vi "Unload Subpanel VI.vi"(8 "error in":errorcluster, 11 "subpanel refnum":refnum<vi>) -> (0 "error out":errorcluster)   [LabVIEW 2010]
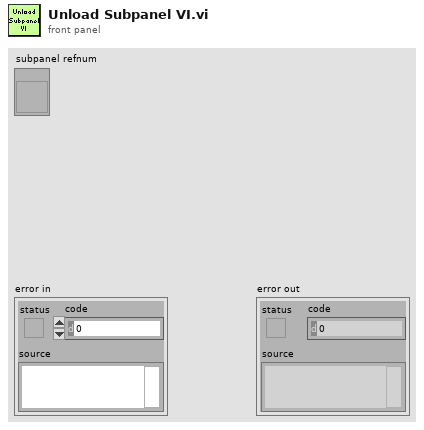
[diagram p1: front panel]
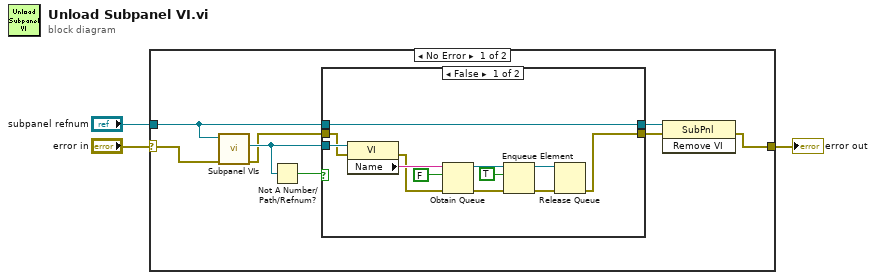
[diagram p0: block diagram]
diagram:
  n1 = case shown="No Error" "error in" {
    selector: "error in" -> [w5 w26]
    tunnel: [w7 w26] -> w2
    tunnel: "subpanel refnum" -> [w10 _]
    frame No Error {
      n2 = call "Subpanel VIs.vi"("error in"=w5, "subpanel refnum"=w10) -> ("error out"=w4:errorcluster, "subpanel VI out"=w6:refnum<vi>)  [unwired: 8 in]
      n3 = Not A Number/Path/Refnum?(number/path/refnum=w6) -> (NaN/Path/Refnum?=w11:bool)
      n4 = case shown="False" w11 {
        tunnel: w10 -> [w23 w25]
        tunnel: [w16 w24] -> w8
        tunnel: [w23 w25] -> w9
        tunnel: w4 -> [w14 w24]
        tunnel: w6 -> [w15 _]
        frame False {
          n5 = property class="VI"(reference=w15, error in=w14) -> (error out=w12:errorcluster, "Name"=w13:string)  [unwired: 1 out]
          n6 = Obtain Queue(name (unnamed)=w13, element data type=FALSE, error in (no error)=w12) -> (queue out=w21:refnum<queue>, error out=w20:errorcluster)  [unwired: 2 in, 1 out]
          n7 = Enqueue Element(queue=w21, element=TRUE, error in (no error)=w20) -> (queue out=w18:refnum<queue>, error out=w17:errorcluster)  [unwired: 1 in, 1 out]
          n8 = Release Queue(queue=w18, error in (no error)=w17) -> (error out=w16:errorcluster)  [unwired: 1 in, 2 out]
        }
        frame True {
        }
      }
      n9 = invoke class="SubPnl" method="Remove VI"(reference=w9, error in=w8) -> (error out=w7:errorcluster)  [unwired: 1 in, 2 out]
    }
    frame Error {
    }
  }
  "error out" <- w2
